vi "Error Display Dialog - no Stop.vi"(0 "Source":string, 5 "Details":string="reason for problem", 7 "dialog type":enum16{"OK message", "Continue or Stop message"}(ring), 9 "Icon to Show":enum16{"Error", "Warning"}(ring), 11 "contname":string="Continue", 12 "stopname":string="Stop") -> (15 "stop event propagated":bool)   [LabVIEW 2015, in "Error Reporting and Storage.lvlib"]
uses:
  <vilib>/Utility/error.llb/ErrWarn.ctl
  <vilib>/event_ctls.llb/eventvkey.ctl
  Error Reporting and Storage.lvlib
panel:
  in  "button 2":string
  out "Source of Error":string
  out "text":string
  out "Error or Warning Glyph":T1=TRUE
  in  "OK":bool
  in  "Stop":bool
  in  "button 1":string
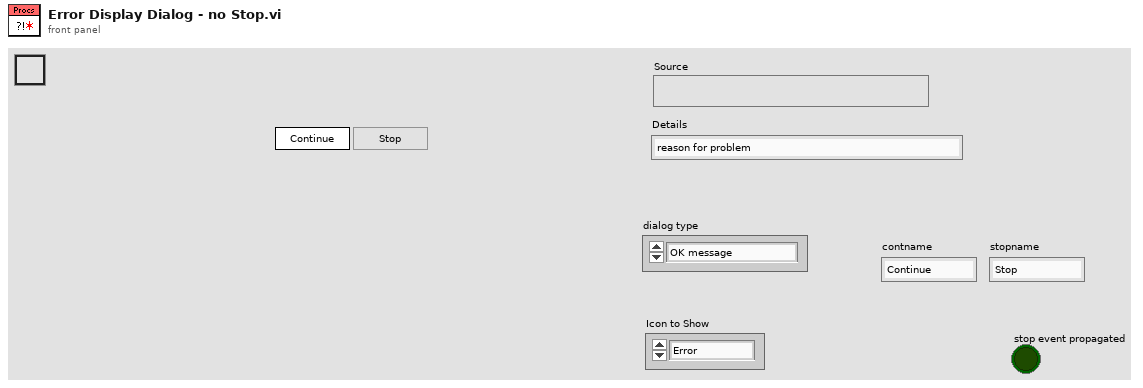
[diagram p1: front panel]
types:
  T1 = typedef "ErrWarn.ctl" = bool
  T2 = enum32{"Invalid", "Standard", "Closed", "Hidden", "Minimized", "Maximized"}
  T3 = cluster{"Control":bool, "Shift":bool, "Key":string}
  T4 = typedef "LVPositionTypeDef.ctl" = cluster{"Left":i32, "Top":i32}
  T5 = typedef "LVRectTypeDef.ctl" = cluster{"Left":i16, "Top":i16, "Right":i16, "Bottom":i16}
  T6 = typedef "eventvkey.ctl" = enum16{"ASCII", "Enter", "Return", "Shift", "Ctrl", "Alt", "Cmd", "Opt", "Caps", "NumLock", "Clear", "Break", "Up", "Down", "Left", "Right", "Insert", "Delete", "Home", "End", "PageUp", "PageDown", "Escape", "Help", "Pause", "ScrollLock", "F1", "F2", "F3", "F4", "F5", "F6", "F7", "F8", "F9", "F10", "F11", "F12", "F13", "F14", "F15", "F16", "F17", "F18", "F19", "F20", "F21", "F22", "F23", "F24", "Play", "VolumeUp", "VolumeDown", "Mute", "Two Byte Char"}
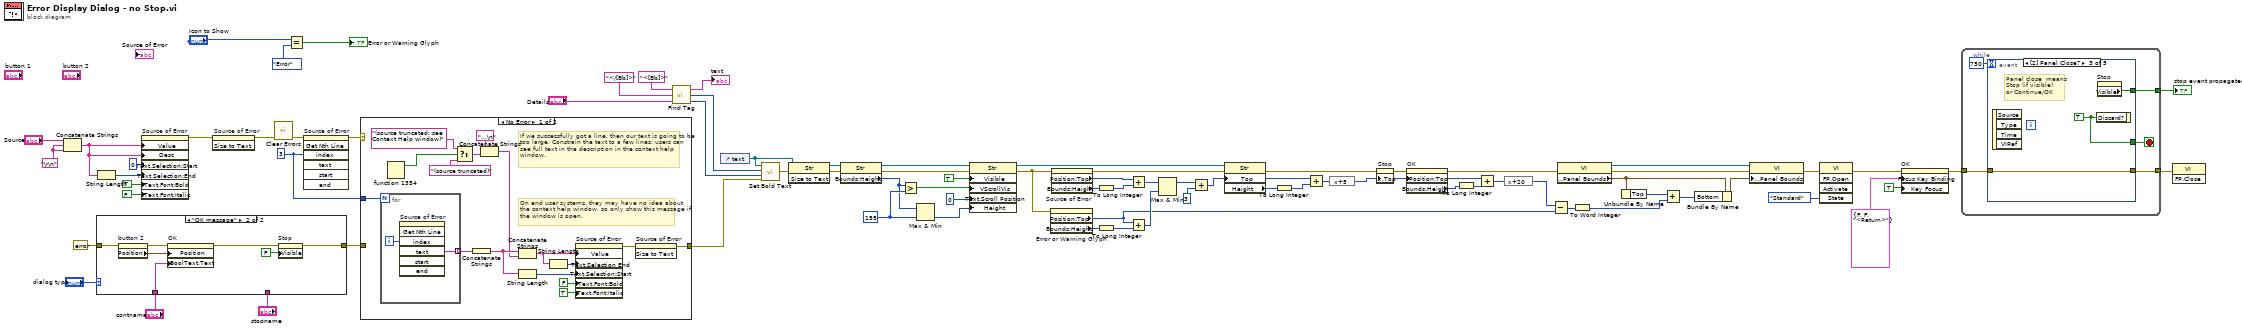
[diagram p0: block diagram]
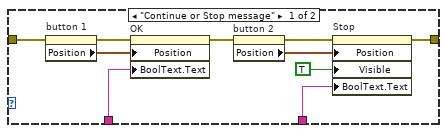
[diagram p2: hidden frame]
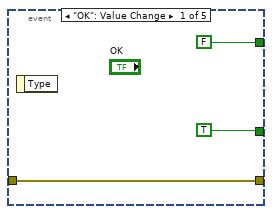
[diagram p3: hidden frame]
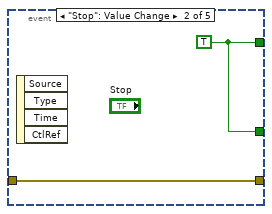
[diagram p4: hidden frame]
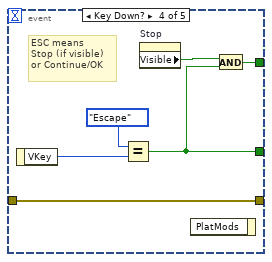
[diagram p5: hidden frame]
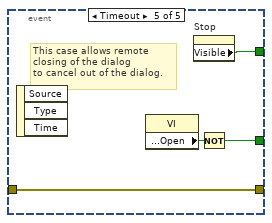
[diagram p6: hidden frame]
diagram:
  w21 = "\r\n"
  w30 = u32 155
  w72 = u32 3 ("index")
  n1 = Concatenate Strings("Source", w21, w21) -> (w17:string)
  n2 = case shown="\"OK message\"" "dialog type" {
    tunnel: "stopname" -> [w90 _]
    tunnel: "contname" -> [w89 w97]
    tunnel: [w82 w91] -> w6
    tunnel: errorcluster {"status"=FALSE, "code"=0, "source"=""} ("error out") -> [w81 w92]
    frame "Continue or Stop message" {
      n3 = property on="button 1" class="Str"(error in=w81) -> (error out=w87:errorcluster, "Position"=w88:T4)  [unwired: 1 in, 1 out]
      n4 = property on="OK" class="Bool"(error in=w87, "Position"=w88, "BoolText.Text"=w89) -> (error out=w85:errorcluster)  [unwired: 1 in, 1 out]
      n5 = property on="button 2" class="Str"(error in=w85) -> (error out=w84:errorcluster, "Position"=w83:T4)  [unwired: 1 in, 1 out]
      n6 = property on="Stop" class="Bool"(error in=w84, "Position"=w83, "Visible"=TRUE, "BoolText.Text"=w90) -> (error out=w82:errorcluster)  [unwired: 1 in, 1 out]
    }
    frame "OK message" {
      n7 = property on="button 2" class="Str"(error in=w92) -> (error out=w95:errorcluster, "Position"=w96:T4)  [unwired: 1 in, 1 out]
      n8 = property on="OK" class="Bool"(error in=w95, "Position"=w96, "BoolText.Text"=w97) -> (error out=w93:errorcluster)  [unwired: 1 in, 1 out]
      n9 = property on="Stop" class="Bool"(error in=w93, "Visible"=FALSE) -> (error out=w91:errorcluster)  [unwired: 1 in, 1 out]
    }
  }
  n10 = String Length(string=w17) -> (length=w69:i32)
  n11 = property on="Source of Error" class="Str"("Value"=w17, "Desc"=w17, "Text.Selection:Start"=u32 0, "Text.Selection:End"=w69, "Text.Font:Bold"=TRUE, "Text.Font:Italic"=FALSE) -> (error out=w71:errorcluster)  [unwired: 2 in, 1 out]
  n12 = invoke on="Source of Error" class="Str" method="Size to Text"(error in=w71) -> (error out=w75:errorcluster)  [unwired: 2 in, 2 out]
  n13 = call <vilib>:"Clear Errors.vi"("error in (no error)"=w75) -> ("error out"=w74:errorcluster)  [unwired: 5 in, 1 out]
  n14 = Equal?(x="Icon to Show", y=enum16{"Error", "Warning"}."Error") -> (x = y?=→"Error or Warning Glyph":bool)
  n15 = invoke on="Source of Error" class="Str" method="Get Nth Line"(error in=w74, "index"=w72) -> (error out=w73:errorcluster)  [unwired: 5 in, 6 out]
  n16 = case shown="No Error" w73 {
    tunnel: w72 -> [w113 _]
    tunnel: [w100 w116] -> w77
    tunnel: w6 -> [_ w116]
    frame No Error {
      # "If we successfully got a line, then our text is going to be too large. Constrain the text to a few lines; users can see full text in the description in the context help window."
      # "On end user systems, they may have no idea about the context help window, so only show this message if the window is open."
      n17 = for {
        N: w113 -> [_]
        tunnel: [w114] -> w112 mode=indexing
        i -> [w115]
        n18 = invoke on="Source of Error" class="Str" method="Get Nth Line"("index"=w115) -> ("text"=w114:string)  [unwired: 6 in, 6 out]
      }
      n19 = fn#1354() -> (1:w106:bool)  [unwired: 1 out]
      n20 = Select(t="(source truncated; see Context Help window)" ("truncated & CH message"), s=w106, f="(source truncated)" ("truncated message")) -> (s? t:f=w104:string)
      n21 = Concatenate Strings(w112) -> (w111:string)
      n22 = Concatenate Strings("...\n" ("string"), w104) -> (w102:string)
      n23 = Concatenate Strings(w111, w102) -> (w98:string)
      n24 = String Length(string=w111) -> (length=w107:i32)
      n25 = String Length(string=w98) -> (length=w99:i32)
      n26 = property on="Source of Error" class="Str"("Value"=w98, "Text.Selection End"=w99, "Text.Selection:Start"=w107, "Text.Font:Bold"=FALSE, "Text.Font:Italic"=TRUE) -> (error out=w108:errorcluster)  [unwired: 2 in, 1 out]
      n27 = invoke on="Source of Error" class="Str" method="Size to Text"(error in=w108) -> (error out=w100:errorcluster)  [unwired: 2 in, 2 out]
    }
    frame Error {
      # "An error at this point means that there is no line to fetch. That's good. We do not want the text getting too large."
    }
  }
  n28 = call <vilib>:"Find Tag.vi"("string"="Details", "close tag"="</[Bb]>" ("don't translate!"), "open tag"="<[Bb]>" ("don't translate!")) -> ("Length"=w26:i32[], "Start"=w27:i32[], "string out"=→"text":string)
  n29 = control-ref of="text"() -> (w63:refnum<vi>)
  n30 = call <vilib>:"Set Bold Text.vi"("error in"=w77, "Length"=w26, "Start"=w27, "text"=w63) -> ("error out"=w64:errorcluster)  [unwired: 2 in]
  n31 = invoke class="Str" method="Size to Text"(reference=w63, error in=w64) -> (reference out=w62:refnum<vi>, error out=w65:errorcluster)  [unwired: 1 in, 1 out]
  n32 = property class="Str"(reference=w62, error in=w65) -> (reference out=w61:refnum<vi>, error out=w66:errorcluster, "Bounds:Height"=w15:u32)
  n33 = Greater?(x=w15, y=w30) -> (0:w79:bool)
  n34 = Max & Min(x=w15, y=w30) -> (min(x,y)=w10:u32)  [unwired: 1 out]
  n35 = property class="Str"(reference=w61, error in=w66, "Visible"=TRUE ("Defer Panel Updates"), "VScrollVis"=w79, "Text.Scroll Position"=u32 0, "Height"=w10) -> (reference out=w8:refnum<vi>, error out=w7:errorcluster)
  n36 = property on="Error or Warning Glyph" class="Bool"(error in=w7) -> ("Position:Top"=w51:i32, "Bounds:Height"=w58:u32)  [unwired: 1 in, 2 out]
  n37 = property on="Source of Error" class="Str"(error in=w7) -> (error out=w44:errorcluster, "Position:Top"=w46:i32, "Bounds:Height"=w45:u32)  [unwired: 1 in, 1 out]
  n38 = To Long Integer(number=w58) -> (32bit integer=w43:i32)
  n39 = To Long Integer(number=w45) -> (32bit integer=w42:i32)
  n40 = Add(x=w46, y=w42) -> (x+y=w60:i32)
  n41 = Add(x=w51, y=w43) -> (x+y=w59:i32)
  n42 = Max & Min(x=w60, y=w59) -> (max(x,y)=w4:i32)  [unwired: 1 out]
  n43 = Add(x=w4, y=3) -> (x+y=w48:i32)
  n44 = property class="Str"(reference=w8, error in=w44, "Top"=w48) -> (error out=w20:errorcluster, "Height"=w36:u32)  [unwired: 1 out]
  n45 = To Long Integer(number=w36) -> (32bit integer=w37:i32)
  n46 = Add(x=w48, y=w37) -> (x+y=w47:i32)
  n47 = expression code="x+5"(w47) -> (w35:i32)
  n48 = property on="Stop" class="Bool"(error in=w20, "Position:Top"=w35) -> (error out=w34:errorcluster)  [unwired: 1 in, 1 out]
  n49 = property on="OK" class="Bool"(error in=w34, "Position:Top"=w35) -> (error out=w40:errorcluster, "Bounds:Height"=w57:u32)  [unwired: 1 in, 1 out]
  n50 = To Long Integer(number=w57) -> (32bit integer=w41:i32)
  n51 = Add(x=w35, y=w41) -> (x+y=w56:i32)
  n52 = expression code="x+20"(w56) -> (w52:i32)
  n53 = Subtract(x=w52, y=w51) -> (x-y=w33:i32)
  n54 = property class="VI"(error in=w40) -> (reference out=w53:refnum<vi>, error out=w54:errorcluster, "Front Panel Window:Panel Bounds"=w50:T5)  [unwired: 1 in]
  n55 = To Word Integer(number=w33) -> (16bit integer=w31:i16)
  n56 = Unbundle By Name(w50) -> ("Top"=w32:i16)
  n57 = Add(x=w32, y=w31) -> (x+y=w49:i16)
  n58 = Bundle By Name(cluster=w50, "Bottom"=w49) -> (w55:T5)
  n59 = property class="VI"(reference=w53, error in=w54, "Front Panel Window:Panel Bounds"=w55) -> (error out=w76:errorcluster)  [unwired: 1 out]
  n60 = invoke class="VI" method="FP.Open"(error in=w76, "State"=T2."Standard") -> (error out=w18:errorcluster)  [unwired: 3 in, 4 out]
  n61 = property on="OK" class="Bool"(error in=w18, "Focus Key Binding"=T3 {"Control"=FALSE, "Shift"=FALSE, "Key"="<Return>"}, "Key Focus"=TRUE) -> (error out=w2:errorcluster)  [unwired: 1 in, 1 out]
  n62 = while {
    tunnel: [w120] -> w80
    tunnel: [w117] -> w1
    tunnel: w2 -> [w118]
    stop <- w121 stop-if-true
    n63 = event shown="[2] Panel Close?" {
      selector: _ -> [_ _ _ _ _]
      dyn-events: _ -> [_ _ _ _ _]
      timeout: 750 -> [_ _ _ _ _]
      tunnel: [TRUE ("Stop") w126 w129 w131 w137] -> w121
      tunnel: [FALSE ("Stop") w126 w128 w134 w139] -> w120
      tunnel: w118 -> [w122 w125 w127 w130 w136]
      tunnel: [w122 w125 w127 w130 w136] -> w117
      event "OK": Value Change {
        n64 = event-data() -> ()  [unwired: 1 in, 1 out]
      }
      event "Stop": Value Change {
        w126 = TRUE
        n65 = event-data() -> ()  [unwired: 1 in, 4 out]
      }
      event Panel Close? {
        w129 = TRUE ("Discard?")
        # "Panel close  means\nStop (if visible)\nor Continue/OK"
        n66 = event-data() -> ()  [unwired: 1 in, 4 out]
        n67 = event-data("Discard?"=w129) -> ()  [unwired: 1 in, 1 out]
        n68 = property on="Stop" class="Bool"() -> ("Visible"=w128:bool)  [unwired: 2 in, 2 out]
      }
      event Key Down? {
        # "ESC means\nStop (if visible)\nor Continue/OK"
        n69 = event-data() -> ("VKey"=w133:T6)  [unwired: 1 in]
        n70 = Equal?(x=eventvkey."Escape", y=w133) -> (x = y?=w131:bool)
        n71 = property on="Stop" class="Bool"() -> ("Visible"=w135:bool)  [unwired: 2 in, 2 out]
        n72 = event-data() -> ()  [unwired: 2 in, 1 out]
        n73 = And(x=w135, y=w131) -> (x .and. y?=w134:bool)
      }
      event Timeout {
        # "This case allows remote\nclosing of the dialog\nto cancel out of the dialog."
        n74 = event-data() -> ()  [unwired: 1 in, 3 out]
        n75 = property class="VI"() -> ("Front Panel Window:Open"=w138:bool)  [unwired: 2 in, 2 out]
        n76 = property on="Stop" class="Bool"() -> ("Visible"=w139:bool)  [unwired: 2 in, 2 out]
        n77 = Not(x=w138) -> (.not. x?=w137:bool)
      }
    }
  }
  "stop event propagated" <- w80
  n78 = invoke class="VI" method="FP.Close"(error in=w1) -> ()  [unwired: 2 in, 3 out]
